vi "8000000000000000...ffffffffffffffff随机秘钥.vi"() -> (3 "私钥 2":string)   [LabVIEW 2020]
panel:
  out "长度 2":i32
  out "字符串 2":string="0000000000000000000000000000000000000000000000007cce5efdaccf6808"
  out "字符串":string
  out "输出数组":bool[](array[boolean])
  out "十六进制整型字符串":string
  out "长度":i32
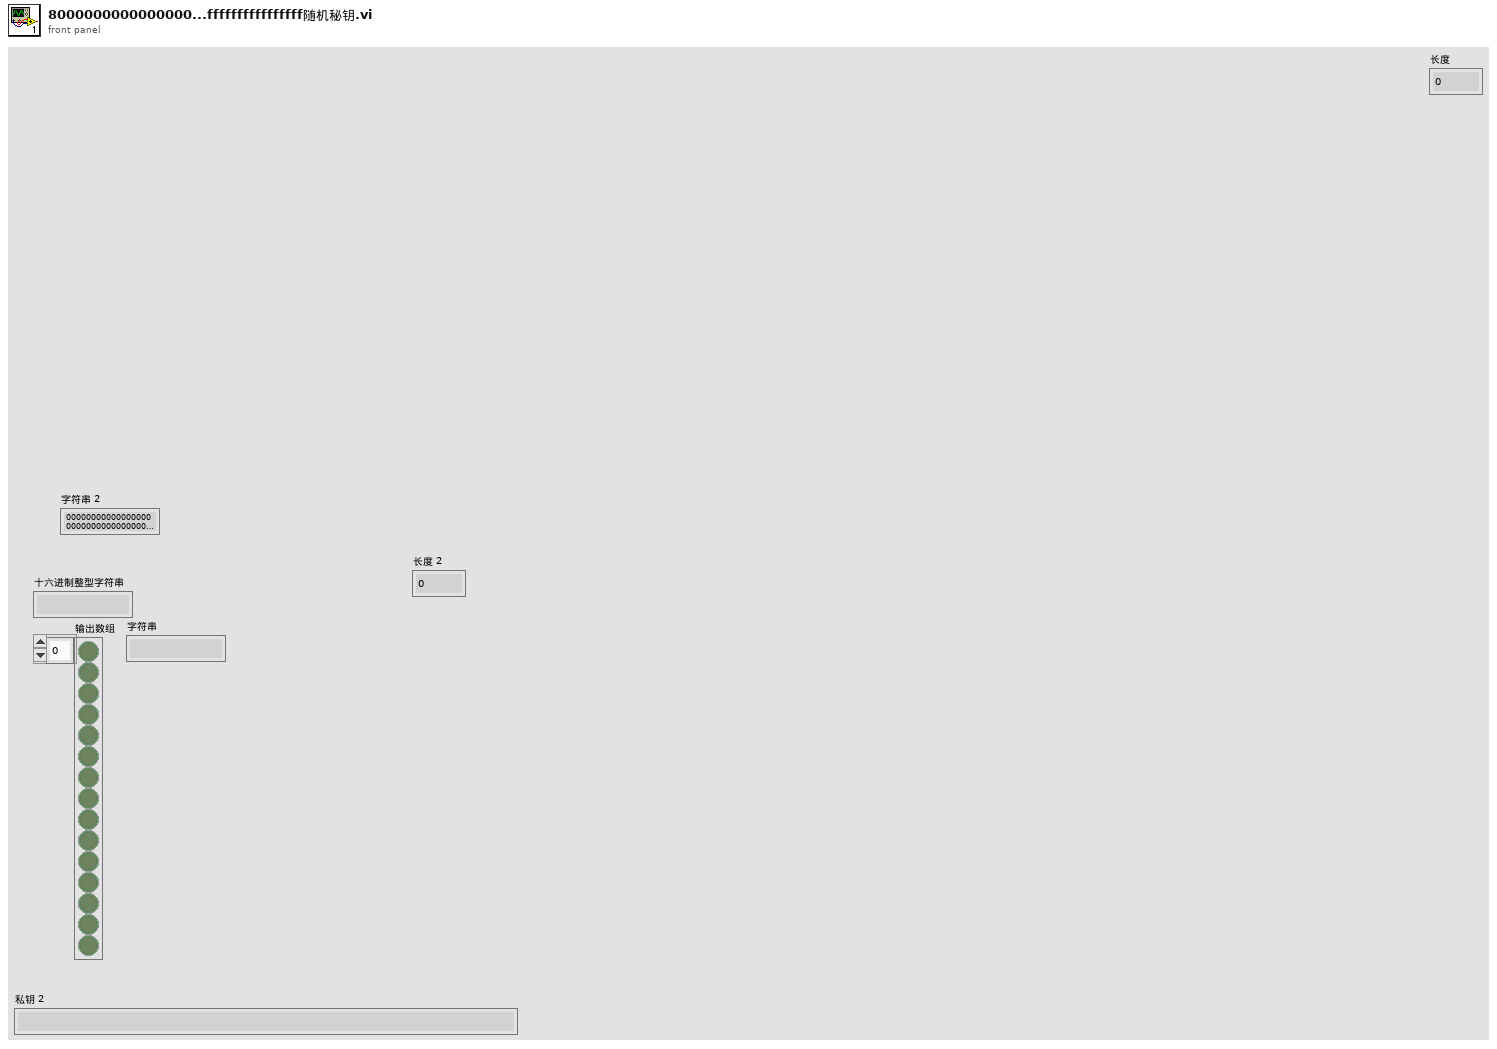
[diagram p1: front panel]
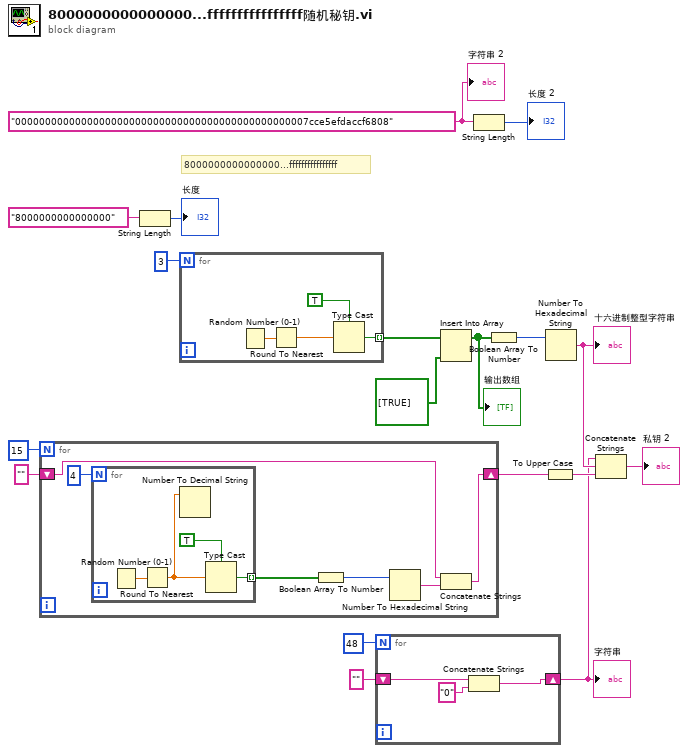
[diagram p0: block diagram]
diagram:
  w3 = "0000000000000000000000000000000000000000000000007cce5efdaccf6808"
  # "8000000000000000...ffffffffffffffff"
  n1 = for {
    N: 15 -> [_]
    shift-right: [w19] -> w16
    shift-left: "" -> [w21]
    n2 = for {
      N: 4 -> [_]
      tunnel: [w25] -> w23 mode=indexing
      n3 = Random Number (0-1)() -> (number: 0 to 1=w28:dbl)
      n4 = Round To Nearest(number=w28) -> (nearest integer value=w27:dbl)
      n5 = Number To Decimal String(number=w27) -> ()  [unwired: 1 in, 1 out]
      n6 = Type Cast(type=TRUE, x=w27) -> (*(type *) &x=w25:bool)
    }
    n7 = Boolean Array To Number(Boolean array=w23) -> (number=w22:u32)
    n8 = Number To Hexadecimal String(2:w22) -> (0:w20:string)  [unwired: 1 in]
    n9 = Concatenate Strings(w21, w20) -> (w19:string)
  }
  n10 = String Length(string="8000000000000000") -> (length=→"长度":i32)
  n11 = for {
    N: 3 -> [_]
    tunnel: [w29] -> w10 mode=indexing
    n12 = Random Number (0-1)() -> (number: 0 to 1=w32:dbl)
    n13 = Round To Nearest(number=w32) -> (nearest integer value=w31:dbl)
    n14 = Type Cast(type=TRUE, x=w31) -> (*(type *) &x=w29:bool)
  }
  n15 = for {
    N: 48 -> [_]
    shift-right: [w33] -> w5
    shift-left: "" -> [w35]
    n16 = Concatenate Strings(w35, "0") -> (w33:string)
  }
  "字符串" <- w5
  n17 = Insert Into Array(array=w10, new element=bool[] [TRUE]) -> (w12:bool[])  [unwired: 1 in]
  "输出数组" <- w12
  n18 = String Length(string=w3) -> (length=→"长度 2":i32)
  n19 = Boolean Array To Number(Boolean array=w12) -> (number=w11:u32)
  n20 = To Upper Case(1:w16) -> (0:w7:string)
  n21 = Number To Hexadecimal String(2:w11) -> (0:w8:string)  [unwired: 1 in]
  "十六进制整型字符串" <- w8
  n22 = Concatenate Strings(w5, w8, w7) -> (→"私钥 2":string)
  "字符串 2" <- w3
